vi "Wysylanie UDP do SbRIO.vi"(7 "Cluster":T2, 10 "output cluster":T1) -> (1 "error out udp":errorcluster, 2 "output cluster 2":T1, 3 "connection ID out":refnum<k16>, 4 "stop error ?":bool)   [LabVIEW 2015]
uses:
  QMH Fundamentals - Message Cluster.ctl
panel:
  out "length":i32
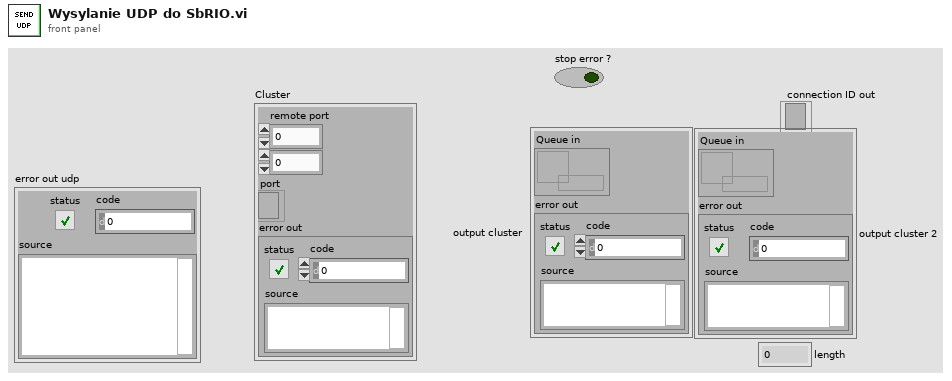
[diagram p1: front panel]
types:
  T1 = cluster{"Queue in":refnum<queue>, "error out":errorcluster}
  T2 = cluster{"remote port":u16, u32, "port":refnum<k16>, "error out":errorcluster}
  T3 = typedef "QMH Fundamentals - Message Cluster.ctl" = cluster{"Message":string, "Message Data":variant}
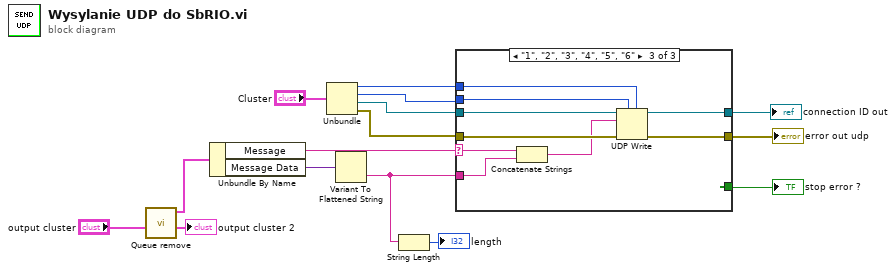
[diagram p0: block diagram]
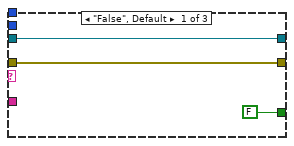
[diagram p2: hidden frame]
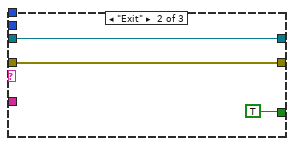
[diagram p3: hidden frame]
diagram:
  n1 = call "Queue remove.vi"("output cluster"="output cluster") -> ("output cluster 2"=→"output cluster 2":T1, "Message Cluster"=w3:T3)  [unwired: 9 in]
  n2 = Unbundle By Name(w3) -> ("Message"=w6:string, "Message Data"=w7:variant)
  n3 = Unbundle("Cluster") -> ("remote port"=w12:u16, w13:u32, "port"=w11:refnum<k16>, "error out"=w10:errorcluster)
  n4 = Variant To Flattened String(Variant=w7) -> (data string=w5:string)  [unwired: 1 out]
  n5 = String Length(string=w5) -> (length=→"length":i32)
  n6 = case shown="\"1\", \"2\", \"3\", \"4\", \"5\", \"6\"" w6 {
    selector: w6 -> [_ _ w22]
    tunnel: w13 -> [_ _ w26]
    tunnel: w12 -> [_ _ w25]
    tunnel: w11 -> [w16 w19 w27]
    tunnel: w10 -> [w18 w21 w30]
    tunnel: [w18 w21 w29] -> w14
    tunnel: [FALSE TRUE _] -> w15
    tunnel: w5 -> [_ _ w23]
    tunnel: [w16 w19 w28] -> w8
    frame "False", Default {
    }
    frame "Exit" {
    }
    frame "1", "2", "3", "4", "5", "6" {
      n7 = Concatenate Strings(w22, w23) -> (w24:string)
      n8 = UDP Write(address=w26, port or service name=w25, connection ID=w27, data in=w24, 8:w30) -> (error out=w29:errorcluster, 3:w28:refnum<k16>)  [unwired: 1 in]
    }
  }
  "stop error ?" <- w15
  "error out udp" <- w14
  "connection ID out" <- w8
